vi "Browse Callback Path.vi"(7 "Parent VI Ref":refnum<vi>, 11 "Init Path in":string) -> (3 "Init Path out":path)   [LabVIEW 2021]
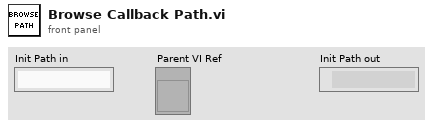
[diagram p1: front panel]
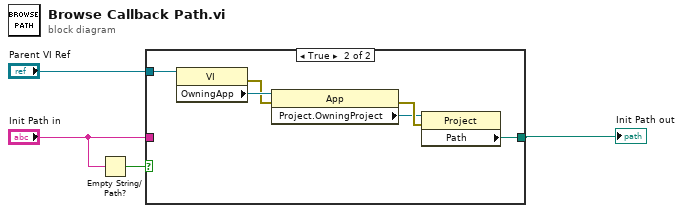
[diagram p0: block diagram]
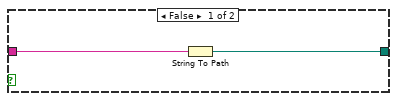
[diagram p2: hidden frame]
diagram:
  n1 = Empty String/Path?(string/path="Init Path in") -> (empty?=w1:bool)
  n2 = case shown="True" w1 {
    tunnel: "Init Path in" -> [w6 _]
    tunnel: [w5 w7] -> w3
    tunnel: "Parent VI Ref" -> [_ w8]
    frame False {
      n3 = String To Path(string=w6) -> (path=w5:path)
    }
    frame True {
      n4 = property class="VI"(reference=w8) -> (error out=w9:errorcluster, "OwningApp"=w10:refnum<vi>)  [unwired: 1 in, 1 out]
      n5 = property class="App"(reference=w10, error in=w9) -> (error out=w12:errorcluster, "Project.OwningProject"=w11:refnum<vi>)  [unwired: 1 out]
      n6 = property class="Project"(reference=w11, error in=w12) -> ("Path"=w7:path)  [unwired: 2 out]
    }
  }
  "Init Path out" <- w3
